vi "EncoderSpeedMise.vi"(8 "error in (no error)":errorcluster, 10 "Encoder 1 Controller":T3={"Sample time (uS)"=300000, "Reset"=FALSE}, 11 "Cluster in":T1={FALSE, "Tick Count(uSec)"=0, "Counter Value"=[0, 0, 0, 0], "x-y"=[0, 0, 0, 0]}) -> (0 "error out":errorcluster, 1 "Updated":bool, 2 "output cluster":T2, 3 "Cluster Out":T1, 4 "Tick Count(uSec)":u32 caption="Tick Count(Ticks)")   [LabVIEW 2018]
uses:
  Downloads/Robotiikka21.12/Robotiikka/Controls/EncoderController.ctl
  <vilib>/myRIO/Common/Instrument Driver Framework/myRIO v1.0/Encoder/typedefs/Encoder Signal Mode.ctl
  <vilib>/myRIO/Instrument Drivers/Onboard IO/Encoder/typedefs/Encoder Reference.ctl
  <vilib>/myRIO/Common/Instrument Driver Framework/Utilities/typedefs/myRIO Generic Hardware Reference.ctl
  <vilib>/myRIO/Common/Instrument Driver Framework/Utilities/typedefs/Hardware Version Enum.ctl
  <vilib>/myRIO/Common/Instrument Driver Framework/Utilities/typedefs/myRIO v1.0 Reference.ctl
  <vilib>/myRIO/Common/Instrument Driver Framework/Utilities/typedefs/Generic FPGA Reference.ctl
  <vilib>/myRIO/Common/Instrument Driver Framework/myRIO v1.0/Encoder/typedefs/Encoder Channels Enum.ctl
  <vilib>/myRIO/Common/Instrument Driver Framework/myRIO v1.0/Encoder/typedefs/Encoder Configuration v1.0.ctl
  <vilib>/userdefined/High Color/nirio_resource_hc.ctl
  <vilib>/myRIO/Common/Instrument Driver Framework/Utilities/vis/Is FPGA Ref Available.vi
  <vilib>/myRIO/Common/Instrument Driver Framework/myRIO v1.0/Encoder/vis/myRIO v1.1 Open Encoder.vi
  <vilib>/myRIO/Instrument Drivers/Onboard IO/Encoder/vis/Read.vi
  <vilib>/myRIO/Common/Instrument Driver Framework/Utilities/vis/Validate Channels.vi
  <vilib>/myRIO/Common/Instrument Driver Framework/myRIO v1.0/Encoder/vis/myRIO v1.0 Reserve Encoder.vi
  <vilib>/myRIO/Common/Instrument Driver Framework/myRIO v1.0/Encoder/vis/myRIO v1.0 Build MUX Configuration Encoder.vi
  <vilib>/myRIO/Common/Instrument Driver Framework/myRIO v1.0/Resource Manager/vis/myRIO v1.0 Reserve Channel List.vi
  <vilib>/myRIO/Common/Instrument Driver Framework/myRIO v1.0/Resource Manager/vis/myRIO v1.0 Create Configuration List.vi
  <vilib>/myRIO/Common/Instrument Driver Framework/myRIO v1.0/Resource Manager/vis/myRIO v1.0 Reserve Channel.vi
  <vilib>/myRIO/Common/Instrument Driver Framework/myRIO v1.0/Resource Manager/vis/myRIO v1.0 Unreserve Channel.vi
  <vilib>/myRIO/Common/Instrument Driver Framework/myRIO v1.0/Resource Manager/vis/myRIO v1.0 Build Mutex Name.vi
  <vilib>/Utility/VariantDataType/GetNumericInfo.vi
  <vilib>/Utility/error.llb/Error Cluster From Error Code.vi
  <vilib>/myRIO/Common/Instrument Driver Framework/myRIO v1.0/myRIO v1.1 Open.vi
  <vilib>/myRIO/Common/Instrument Driver Framework/Utilities/vis/IO Manager.vi
  <vilib>/myRIO/Common/Instrument Driver Framework/Utilities/vis/Configuration Manager.vi
  <vilib>/myRIO/Common/Instrument Driver Framework/myRIO v1.0/Resource Manager/vis/myRIO v1.0 Configure IO.vi
  <vilib>/myRIO/Common/Instrument Driver Framework/myRIO v1.0/myRIO v1.0 Close.vi
  <vilib>/myRIO/Common/Instrument Driver Framework/myRIO v1.0/Encoder/vis/myRIO v1.0 Configure Encoder.vi
  <vilib>/myRIO/Common/Instrument Driver Framework/myRIO v1.0/Encoder/vis/myRIO v1.0 Read Encoder.vi
  <vilib>/myRIO/Express VI/Onboard IO/Encoder/Encoder Express VI.xnode
  <vilib>/myRIO/Instrument Drivers/Onboard IO/Encoder/vis/myRIO Encoder Open.xnode
  <vilib>/myRIO/Common/Instrument Driver Framework/myRIO v1.0/Encoder/typedefs/Encoder Count Direction Enum.ctl
  <vilib>/rvi/Arithmetic/AddSubMult/XNode/nirviSatArithmetic.xnode
  <vilib>/myRIO/Instrument Drivers/Onboard IO/Encoder/Encoder.lvlib
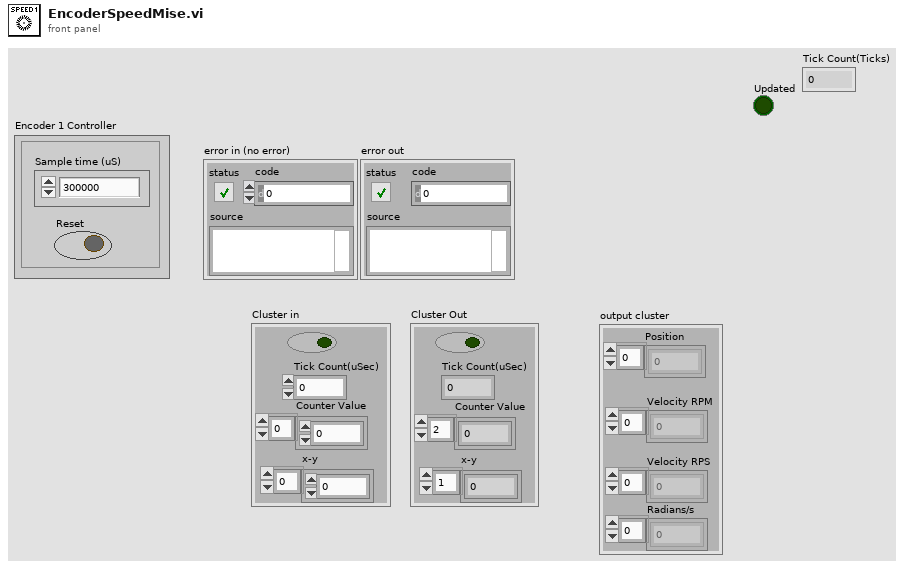
[diagram p1: front panel]
types:
  T1 = cluster{bool, "Tick Count(uSec)":u32, "Counter Value":i32[], "x-y":i32[]}
  T2 = cluster{"Position":i32[], "Velocity RPM":dbl[], "Velocity RPS":dbl[], "Radians/s":dbl[]}
  T3 = typedef "EncoderController.ctl" = cluster{"Sample time (uS)":u32, "Reset":bool}
  T4 = cluster{"Counter Value":i32[], dbl[], dbl[], dbl[]}
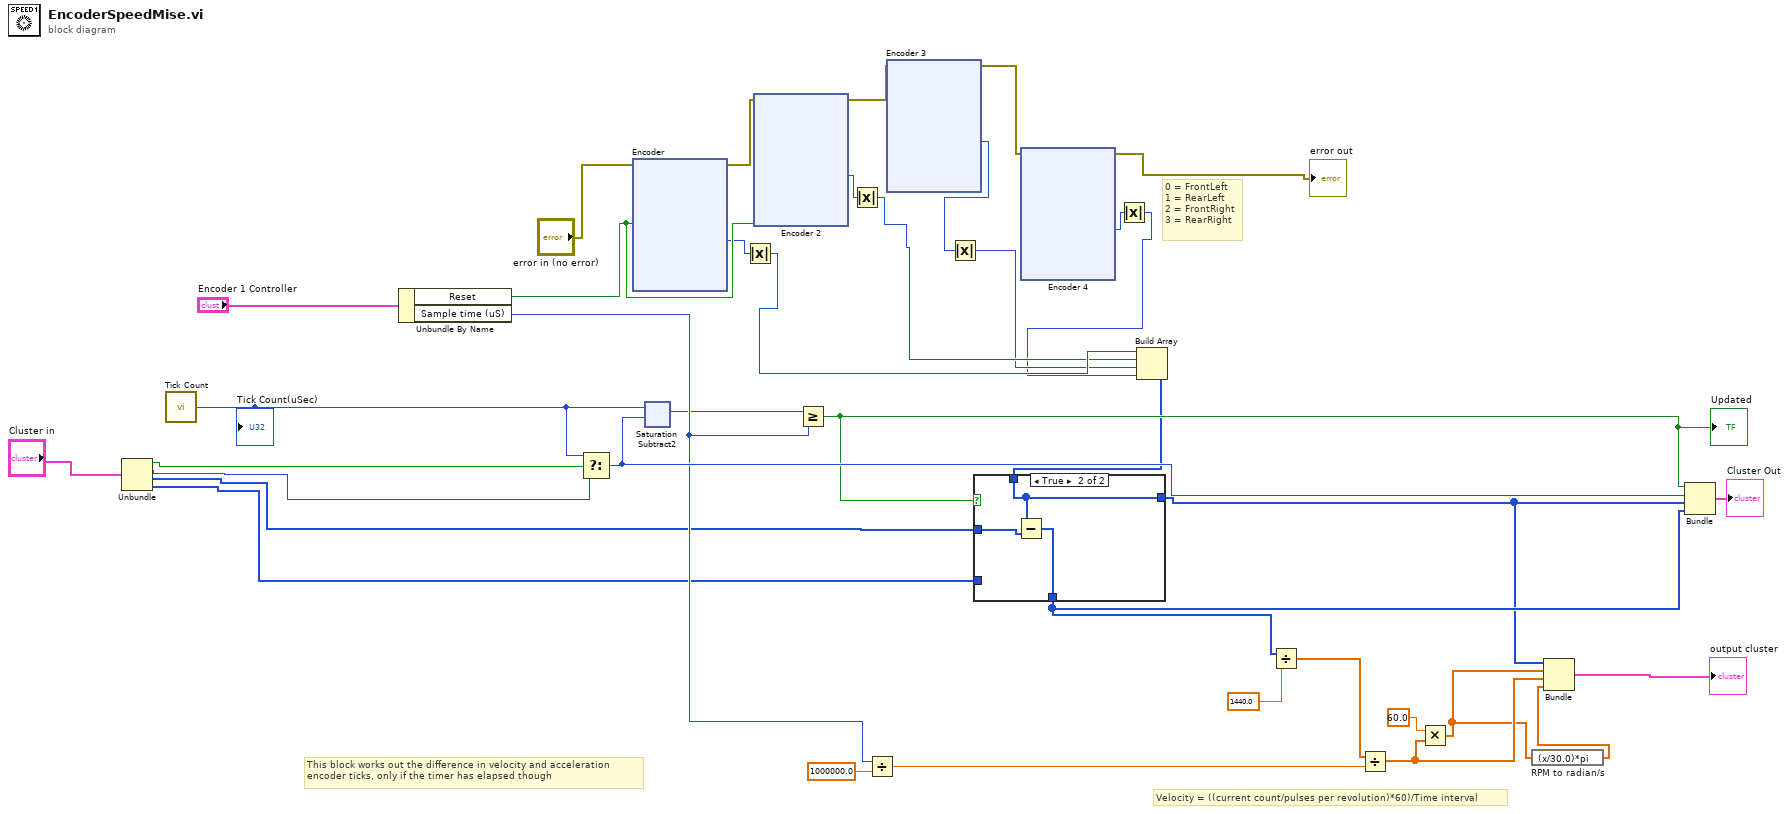
[diagram p0: block diagram]
diagram:
  # "0 = FrontLeft\n1 = RearLeft\n2 = FrontRight\n3 = RearRight"
  # "Velocity = ((current count/pulses per revolution)*60)/Time interval"
  # "This block works out the difference in velocity and acceleration \nencoder ticks, only if the timer has elapsed though"
  n1 = Unbundle("Cluster in") -> (w19:bool, "Tick Count(uSec)"=w18:u32, "Counter Value"=w17:i32[], "x-y"=w16:i32[])
  n2 = call "Tick Count"() -> ("Tick Count(uSec)"=w30:u32)
  "Tick Count(uSec)" <- w30
  n3 = Unbundle By Name("Encoder 1 Controller") -> ("Reset"=w12:bool, "Sample time (uS)"=w27:u32)
  n4 = Select(t=w30, s=w19, f=w18) -> (s? t:f=w29:u32)
  n5 = xnode "Encoder"("Reset Counter"=w12, "error in (no error)"="error in (no error)") -> ("Counter Value"=w8:i32, "error out"=w23:errorcluster)  [unwired: 2 out]
  n6 = xnode ("Saturation Subtract2")("x"=w30, "y"=w29) -> ("x-y"=w24:u32)
  n7 = Absolute Value(x=w8) -> (abs(x)=w7:i32)
  n8 = xnode "Encoder 2"("Reset Counter"=w12, "error in (no error)"=w23) -> ("Counter Value"=w6:i32, "error out"=w11:errorcluster)  [unwired: 2 out]
  n9 = Greater Or Equal?(x=w24, y=w27) -> (x >= y?=w28:bool)
  "Updated" <- w28
  n10 = Absolute Value(x=w6) -> (abs(x)=w5:i32)
  n11 = Divide(x=w27, y=1000000.0) -> (x/y=w33:dbl)
  n12 = xnode "Encoder 3"("error in (no error)"=w11) -> ("Counter Value"=w4:i32, "error out"=w10:errorcluster)  [unwired: 1 in, 2 out]
  n13 = Absolute Value(x=w4) -> (abs(x)=w3:i32)
  n14 = xnode "Encoder 4"("error in (no error)"=w10) -> ("Counter Value"=w1:i32, "error out"=→"error out":errorcluster)  [unwired: 1 in, 2 out]
  n15 = Absolute Value(x=w1) -> (abs(x)=w2:i32)
  n16 = Build Array(w7, w5, w3, w2) -> (w22:i32[])
  n17 = case shown="True" w28 {
    tunnel: w17 -> [w39 w43]
    tunnel: [w40 w42] -> w34
    tunnel: w16 -> [w40 _]
    tunnel: [w39 w41] -> w32
    tunnel: w22 -> [_ w41]
    frame False {
    }
    frame True {
      n18 = Subtract(x=w41, y=w43) -> (x-y=w42:i32[])
    }
  }
  n19 = Divide(x=w34, y=1440.0) -> (x/y=w35:dbl[])
  n20 = Divide(x=w35, y=w33) -> (x/y=w36:dbl[])
  n21 = Multiply(x=60.0 ("y"), y=w36) -> (x*y=w15:dbl[])
  n22 = expression code="(x/30.0)*pi" "RPM to radian/s"(w15) -> (w14:dbl[])
  n23 = Bundle("Counter Value"=w32, w15, w36, w14) -> (→"output cluster":T4)  [unwired: 1 in]
  n24 = Bundle(w28, "Tick Count(uSec)"=w29, "Counter Value"=w32, "x-y"=w34) -> (→"Cluster Out":T1)  [unwired: 1 in]
